vi "make_waveform (SubVI).vi"(6 "dt":dbl, 9 "Array":dbl[](array[numeric])) -> (1 "output waveform 3":waveform(dbl), 2 "output waveform 2":waveform(dbl), 3 "output waveform":waveform(dbl))   [LabVIEW 2021]
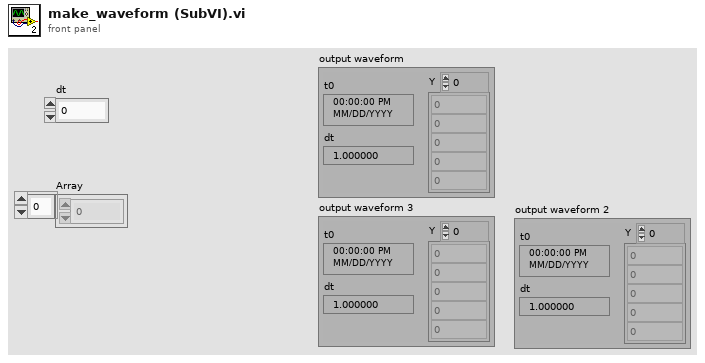
[diagram p1: front panel]
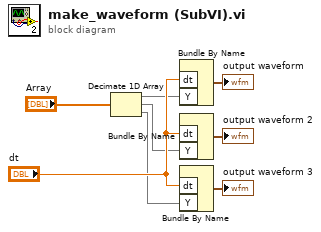
[diagram p0: block diagram]
diagram:
  n1 = Decimate 1D Array("Array") -> (w4:dbl[], w6:dbl[], w7:dbl[])
  n2 = Bundle By Name("dt"="dt", "Y"=w4) -> (→"output waveform":waveform(dbl))  [unwired: 1 out]
  n3 = Bundle By Name("dt"="dt", "Y"=w6) -> (→"output waveform 2":waveform(dbl))  [unwired: 1 out]
  n4 = Bundle By Name("dt"="dt", "Y"=w7) -> (→"output waveform 3":waveform(dbl))  [unwired: 1 out]
